vi "Main.vi"(11 "Script in":refnum<class "Script.lvclass">) -> ()   [LabVIEW 2021, in "_Template.lvlib" / "Script.lvlib" / "Script.lvclass"]
uses:
  Script.lvclass
  Script.lvclass/Script.ctl
  Script.lvlib
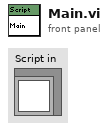
[diagram p1: front panel]
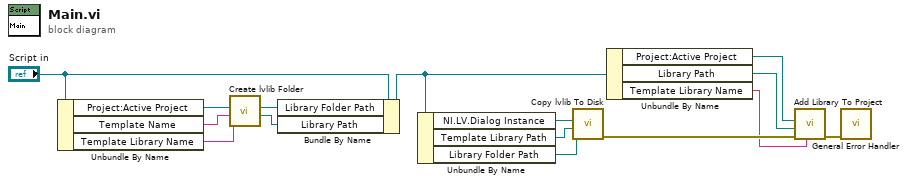
[diagram p0: block diagram]
diagram:
  n1 = Unbundle By Name("Script in") -> ("Project:Active Project"=w15:refnum<vi>, "Template Name"=w3:string, "Template Library Name"=w2:string)
  n2 = call "Create lvlib Folder.vi"("Template Library Name"=w2, "Template Name"=w3, "Project:Active Project"=w15) -> ("Library Path"=w7:path, "Library Folder Path"=w14:path)  [unwired: 7 in]
  n3 = Bundle By Name(cluster="Script in", "Library Folder Path"=w14, "Library Path"=w7) -> (w6:refnum<class "Script.lvclass">)
  n4 = Unbundle By Name(w6) -> ("NI.LV.Dialog Instance"=w12:refnum<vi>, "Template Library Path"=w11:path, "Library Folder Path"=w10:path)
  n5 = call "Copy lvlib To Disk.vi"("Library Folder Path"=w10, "Template Library Path"=w11, "NI.LV.Dialog Instance"=w12) -> ("error out"=w9:errorcluster)  [unwired: 8 in]
  n6 = Unbundle By Name(w6) -> ("Project:Active Project"=w13:refnum<vi>, "Library Path"=w4:path, "Template Library Name"=w1:string)
  n7 = call "Add Library To Project.vi"("Template Library Name"=w1, "error in"=w9, "Library Path"=w4, "Project:Active Project"=w13) -> ("error out"=w5:errorcluster)  [unwired: 7 in]
  n8 = call <vilib>:"General Error Handler.vi"("error in (no error)"=w5) -> ()  [unwired: 10 in, 5 out]
